vi "SQLite Platform DB Path.vi"(11 "名称或相对路径":string="database1.db") -> (3 "Path out":string)   [LabVIEW 2016, in "SQLite Lib.lvlib"]
uses:
  SQLite Lib.lvlib
  <vilib>/Utility/sysdir.llb/System Directory Type.ctl
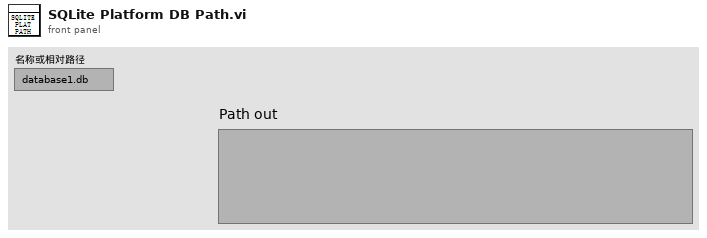
[diagram p1: front panel]
types:
  T1 = typedef "System Directory Type.ctl" = i32
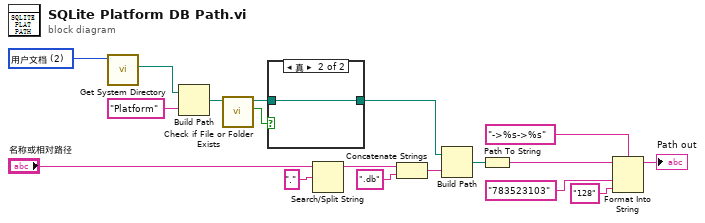
[diagram p0: block diagram]
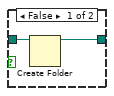
[diagram p2: hidden frame]
diagram:
  w10 = T1 2 items=["用户目录"=0, "用户桌面"=1, "用户文档"=2, "用户应用程序数据"=3, "用户设置"=4, "用户临时目录"=5, "公共文档"=6, "公共应用程序数据"=7, "公共设置"=8, "公共缓存"=13, "系统核心库"=9, "系统安装库"=10, "应用程序文件"=11, "启动盘根目录"=12] ("system directory type")
  n1 = call <vilib>:"Get System Directory.vi"("system directory type"=w10) -> ("system directory"=w9:path)  [unwired: 10 in]
  n2 = Build Path(base path=w9, name or relative path="Platform" ("名称或相对路径")) -> (appended path=w7:path)
  n3 = call <vilib>:"Check if File or Folder Exists.vi"("path"=w7) -> ("file or folder exists?"=w18:bool, "dup path"=w17:path)  [unwired: 8 in, 1 out]
  n4 = case shown="真" w18 {
    tunnel: w17 -> [w20 w21]
    tunnel: [w19 w21] -> w16
    frame False {
      n5 = Create Folder(path (use dialog)=w20) -> (created path=w19:path)  [unwired: 2 in, 2 out]
    }
    frame True {
    }
  }
  n6 = Search/Split String(string="名称或相对路径", search string/char (-)="." ("搜索字符串/字符(-)")) -> (substring before match=w15:string)  [unwired: 1 in, 2 out]
  n7 = Concatenate Strings(w15, ".db" ("字符串")) -> (w11:string)
  n8 = Build Path(base path=w16, name or relative path=w11) -> (appended path=w6:path)
  n9 = Path To String(path=w6) -> (string=w3:string)
  n10 = Format Into String(format string="->%s->%s", initial string=w3, "783523103" ("Enter Password"), "128" ("输入 2")) -> (resulting string=→"Path out":string)  [unwired: 1 in, 1 out]
